vi "Демультиплексор(1-разрядный операнд, 4 выхода).vi"(0 "a":bool, 1 "c":cluster{"c0":bool, "c1":bool}) -> (2 "r0":bool, 3 "r1":bool, 4 "r2":bool, 5 "r3":bool)   [LabVIEW 2013]
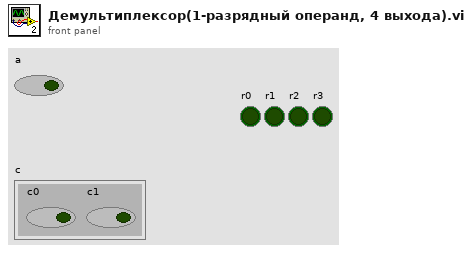
[diagram p1: front panel]
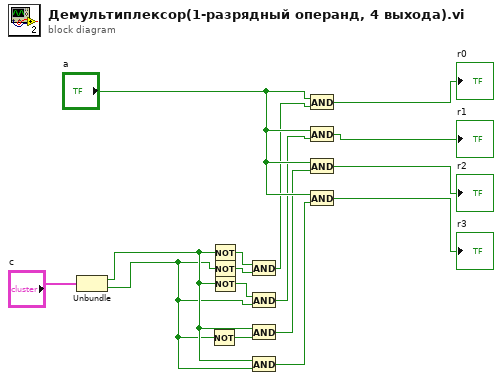
[diagram p0: block diagram]
diagram:
  n1 = Unbundle("c") -> ("c0"=w8:bool, "c1"=w6:bool)
  n2 = Not(x=w6) -> (.not. x?=w7:bool)
  n3 = Not(x=w8) -> (.not. x?=w11:bool)
  n4 = Not(x=w6) -> (.not. x?=w10:bool)
  n5 = Not(x=w8) -> (.not. x?=w9:bool)
  n6 = And(x=w11, y=w10) -> (x .and. y?=w4:bool)
  n7 = And(x=w9, y=w6) -> (x .and. y?=w3:bool)
  n8 = And(x=w8, y=w7) -> (x .and. y?=w2:bool)
  n9 = And(x=w8, y=w6) -> (x .and. y?=w1:bool)
  n10 = And(x="a", y=w4) -> (x .and. y?=→"r0":bool)
  n11 = And(x="a", y=w3) -> (x .and. y?=→"r1":bool)
  n12 = And(x="a", y=w2) -> (x .and. y?=→"r2":bool)
  n13 = And(x="a", y=w1) -> (x .and. y?=→"r3":bool)
